vi "MoveNumericToCell.vi"(6 "Data":string[][](array[string]), 8 "error in (no error)":errorcluster, 9 "Numeric":refnum<vi>, 10 "Cell Position":T1, 11 "Listbox":refnum<vi>) -> (0 "error out":errorcluster)   [LabVIEW 2015, in "Protection and Rolling Counter Addon System Explorer.lvlib"]
uses:
  Protection and Rolling Counter Addon System Explorer.lvlib
  <vilib>/Utility/miscctls.llb/LVRowAndColumnTypeDef.ctl
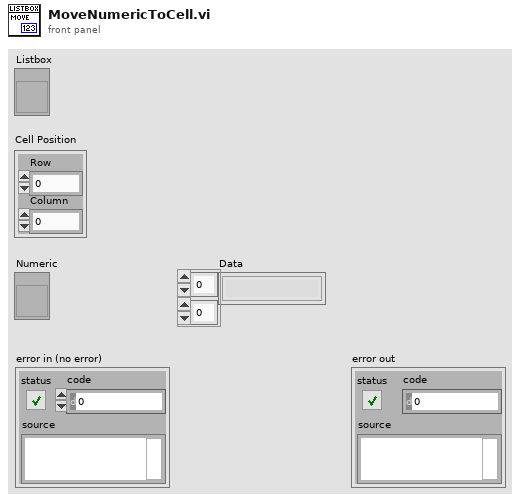
[diagram p1: front panel]
types:
  T1 = typedef "LVRowAndColumnTypeDef.ctl" = cluster{"Row":i32, "Column":i32}
  T2 = typedef "LVBoundsTypeDef.ctl" = cluster{"Width":u32, "Height":u32}
  T3 = typedef "LVPositionTypeDef.ctl" = cluster{"Left":i32, "Top":i32}
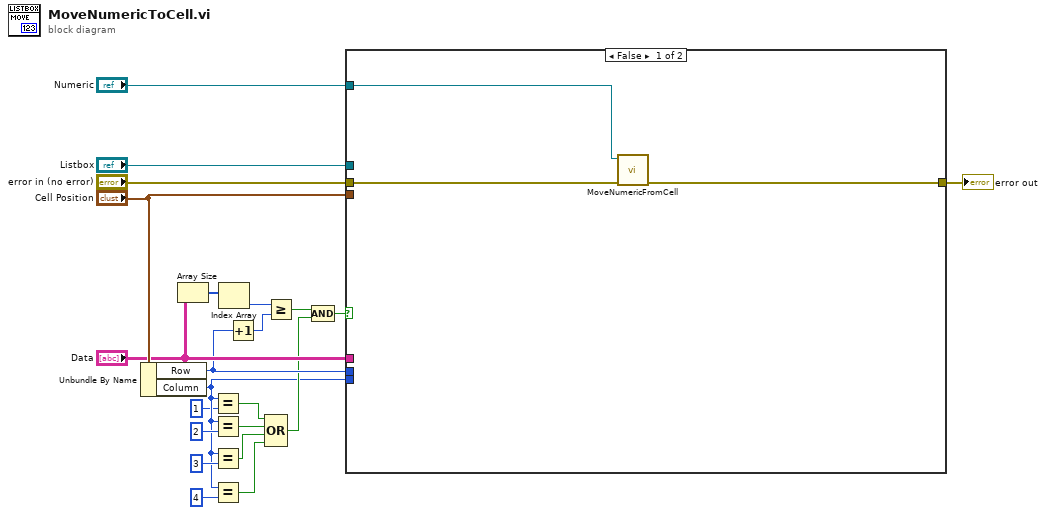
[diagram p0: block diagram]
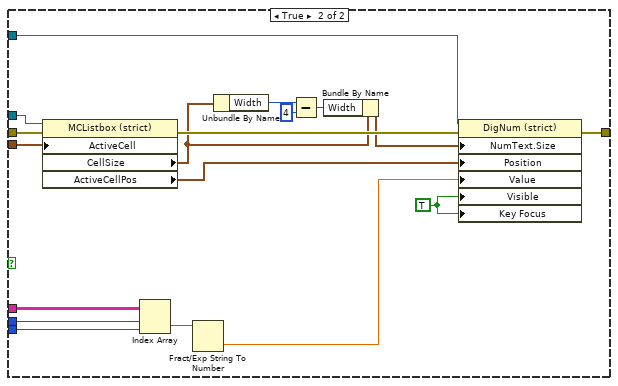
[diagram p2: hidden frame]
diagram:
  n1 = Unbundle By Name("Cell Position") -> ("Row"=w13:i32, "Column"=w2:i32)
  n2 = Array Size(array="Data") -> (size(s)=w16:i32[])
  n3 = Equal?(x=w2, y=1) -> (x = y?=w3:bool)
  n4 = Equal?(x=w2, y=2) -> (x = y?=w7:bool)
  n5 = Equal?(x=w2, y=3) -> (x = y?=w6:bool)
  n6 = Equal?(x=w2, y=4) -> (x = y?=w5:bool)
  n7 = Index Array(array=w16) -> (element=w15:i32)  [unwired: 1 in]
  n8 = Increment(x=w13) -> (x+1=w11:i32)
  n9 = Compound Arithmetic op=OR(w3, w7, w6, w5) -> (w4:bool)
  n10 = Greater Or Equal?(x=w15, y=w11) -> (x >= y?=w14:bool)
  n11 = Compound Arithmetic op=AND(w14, w4) -> (w12:bool)
  n12 = case shown="False" w12 {
    tunnel: "Listbox" -> [_ w43]
    tunnel: "Numeric" -> [w25 w42]
    tunnel: "error in (no error)" -> [w24 w41]
    tunnel: [w23 w39] -> w19
    tunnel: "Cell Position" -> [_ w38]
    tunnel: w13 -> [_ w37]
    tunnel: w2 -> [_ w36]
    tunnel: "Data" -> [_ w26]
    frame False {
      n13 = call "MoveNumericFromCell.vi"("error in (no error)"=w24, "Digital in"=w25) -> ("error out"=w23:errorcluster)  [unwired: 9 in]
    }
    frame True {
      w33 = TRUE ("Visible")
      n14 = property class="MCListbox (strict)"(reference=w43, error in=w41, "ActiveCell"=w38) -> (error out=w40:errorcluster, "CellSize"=w29:T2, "ActiveCellPos"=w32:T3)  [unwired: 1 out]
      n15 = Index Array(array=w26, index (row)=w37, index (col)=w36) -> (element=w35:string)
      n16 = Fract/Exp String To Number(string=w35) -> (number=w34:dbl)  [unwired: 3 in, 1 out]
      n17 = Unbundle By Name(w29) -> ("Width"=w31:u32)
      n18 = Subtract(x=w31, y=u32 4) -> (x-y=w27:u32)
      n19 = Bundle By Name(cluster=w29, "Width"=w27) -> (w28:T2)
      n20 = property class="DigNum (strict)"(reference=w42, error in=w40, "NumText.Size"=w28, "Position"=w32, "Value"=w34, "Visible"=w33, "Key Focus"=w33) -> (error out=w39:errorcluster)  [unwired: 1 out]
    }
  }
  "error out" <- w19
